vi "byte array to number.vi"(9 "Byte Array":u8[](array[numeric]), 10 "Byte Length":u8, 11 "Start Value":u32) -> (1 "Number":u32)   [LabVIEW 2017]
doc: "This VI is used to convert a number stored as a byte array into a single numeric value."
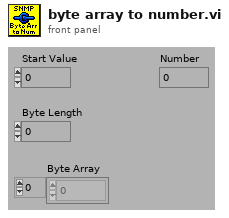
[diagram p1: front panel]
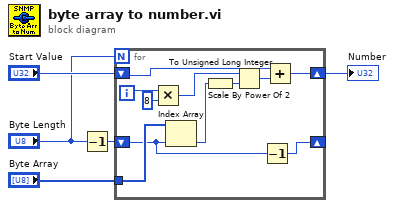
[diagram p0: block diagram]
diagram:
  n1 = Decrement(x="Byte Length") -> (x-1=w2:u8)
  n2 = for {
    N: "Byte Length" -> [_]
    tunnel: "Byte Array" -> [w16]
    shift-right: [w9] -> w1
    shift-left: "Start Value" -> [w7]
    shift-right: [w14] -> _
    shift-left: w2 -> [w15]
    i -> [w13]
    n3 = Multiply(x=w13, y=8) -> (x*y=w11:i32)
    n4 = Index Array(array=w16, index=w15) -> (element=w10:u8)
    n5 = To Unsigned Long Integer(number=w10) -> (unsigned 32bit integer=w6:u32)
    n6 = Scale By Power Of 2(n=w11, x=w6) -> (x*2^n=w8:u32)
    n7 = Decrement(x=w15) -> (x-1=w14:u8)
    n8 = Add(x=w7, y=w8) -> (x+y=w9:u32)
  }
  "Number" <- w1
